vi "20211015_05.vi"() -> ()   [LabVIEW 2019]
panel:
  out "Numeric":i32
  in  "Tab Control":enum32{"Page 1", "Page 2", "Page 3"}(tab)
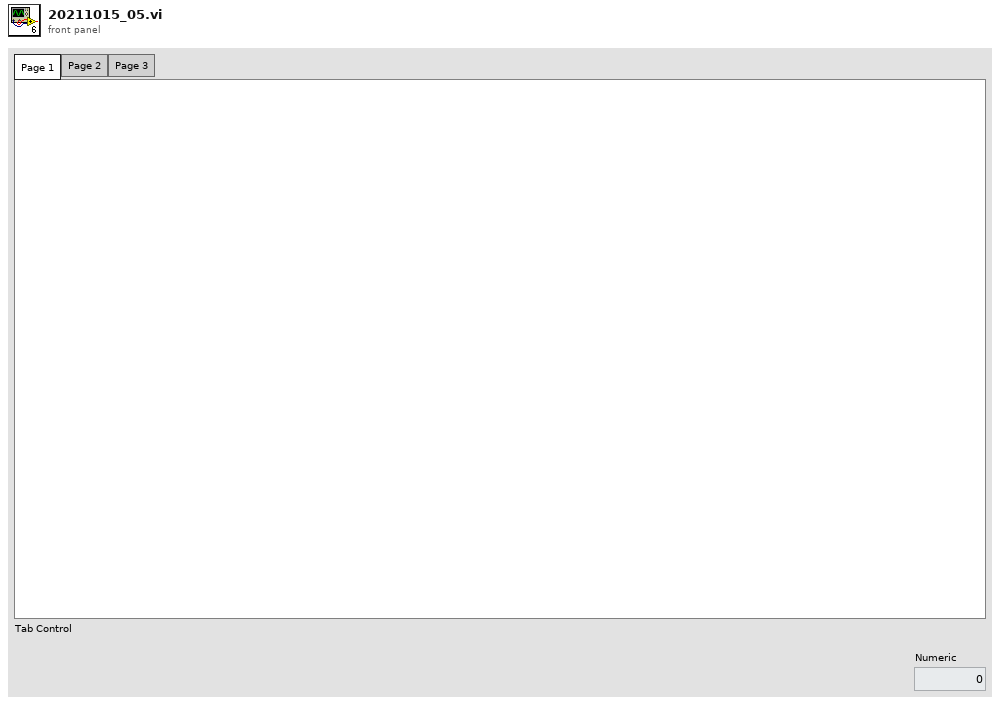
[diagram p1: front panel]
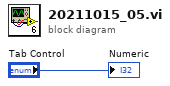
[diagram p0: block diagram]
diagram:
  "Numeric" <- "Tab Control"
